vi "Unflatten UIP Value.vi"(10 "String Value":string, 11 "UIP In":refnum<class "UIP.lvclass">) -> (0 "Error Out":errorcluster, 3 "UIP Out":refnum<class "UIP.lvclass">)   [LabVIEW 2015, in "UIP.lvclass"]
doc: "Overwrite this abstract method to implement child behavior for unflattening the UIP private data from XML compatible string format."
uses:
  UIP.lvclass
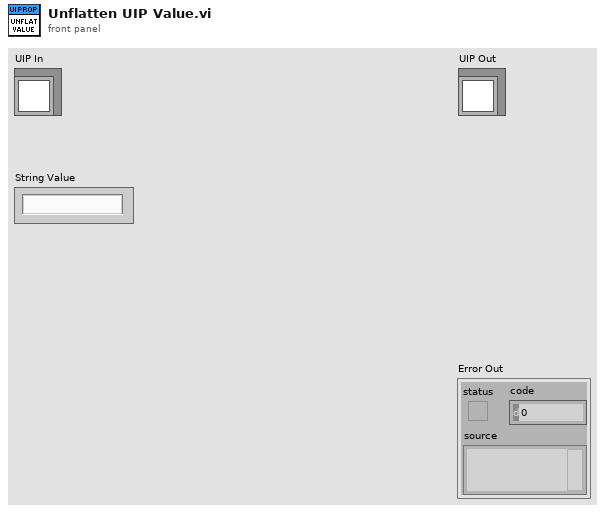
[diagram p1: front panel]
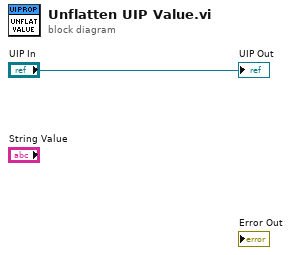
[diagram p0: block diagram]
diagram:
  "UIP Out" <- "UIP In"
